vi "Scripting_RenameClassControlsOfClass.vi"(8 "error in (no error)":errorcluster, 10 "ClassControlName":string, 11 "LVClassLibrary in":refnum<vi>) -> (0 "error out":errorcluster)   [LabVIEW 2020, in "Scripting.lvclass"]
uses:
  <resource>/Framework/Providers/Open_GDS/ClassProviders/Common/ScriptingFunctions/Scripting.lvclass
  <vilib>/regexp/Match Regular Expression.xnode
panel:
  # "<ClassName> in/out\n<ClassName>\nobject in/out\nreference in/out"
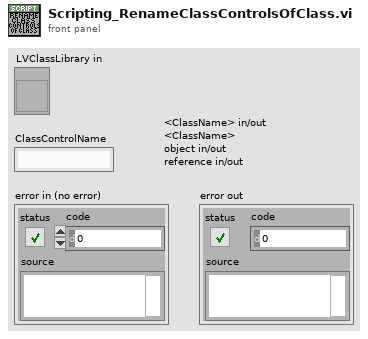
[diagram p1: front panel]
types:
  T1 = enum32{"invalid VI type", "Standard VI", "Control VI", "Global VI", "Polymorphic VI", "Configuration VI", "SubSystem", "Facade VI", "Method VI", "Statechart Diagram VI"}
  T2 = typedef "LVRectTypeDef.ctl" = cluster{"Left":i16, "Top":i16, "Right":i16, "Bottom":i16}
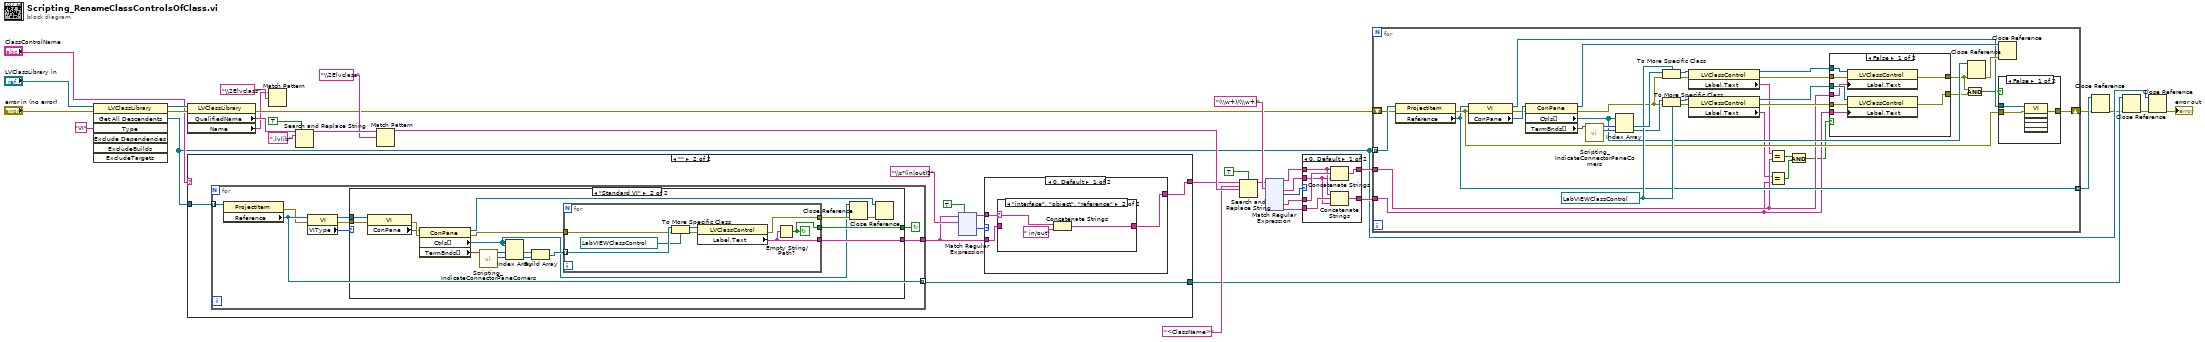
[diagram p0: block diagram]
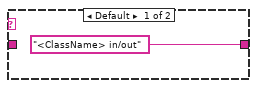
[diagram p3: hidden frame]
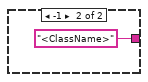
[diagram p4: hidden frame]
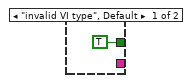
[diagram p5: hidden frame]
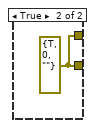
[diagram p7: hidden frame]
diagram:
  n1 = invoke class="LVClassLibrary" method="Get All Descendents"(reference="LVClassLibrary in", error in="error in (no error)", "Type"="VI") -> (reference out=w32:refnum<vi>, error out=w12:errorcluster, "All Descendents"=w8:refnum<vi>[])  [unwired: 4 in, 4 out]
  n2 = property class="LVClassLibrary"(reference=w32, error in=w12) -> (error out=w11:errorcluster, "QualifiedName"=w29:string, "Name"=w1:string)  [unwired: 1 out]
  n3 = case shown="\"\"" "ClassControlName" {
    selector: "ClassControlName" -> [w35 _]
    tunnel: [w35 w39] -> w9
    tunnel: w8 -> [_ w43]
    tunnel: [_ w42] -> w5
    frame Default {
    }
    frame "" {
      n4 = for {
        tunnel: w43 -> [w173] mode=indexing
        tunnel: [w172] -> w36
        tunnel: [w170] -> w42 mode=indexing
        stop <- w171 continue-if-true
        n5 = property class="ProjectItem"(reference=w173) -> (error out=w168:errorcluster, "Reference"=w170:refnum<vi>)  [unwired: 1 in, 1 out]
        n6 = property class="VI"(reference=w170, error in=w168) -> (reference out=w169:refnum<vi>, error out=w167:errorcluster, "VIType"=w166:T1)
        n7 = case shown="\"Standard VI\"" w166 {
          tunnel: [_ w182] -> w172
          tunnel: [TRUE w181] -> w171
          tunnel: w169 -> [_ w176]
          tunnel: w167 -> [_ w175]
          frame "invalid VI type", Default {
          }
          frame "Standard VI" {
            n8 = property class="VI"(reference=w176, error in=w175) -> (error out=w191:errorcluster, "ConPane"=w187:refnum<vi>)  [unwired: 1 out]
            n9 = property class="ConPane"(reference=w187, error in=w191) -> (reference out=w177:refnum<vi>, error out=w183:errorcluster, "Ctrls[]"=w179:refnum<vi>[], "TermBnds[]"=w188:T2[])
            n10 = call <resource>:"Scripting_IndicateConnectorPaneCorners.vi"("TermBnds[]"=w188) -> ("RightTop"=w190:i32, "LeftTop"=w189:i32)  [unwired: 7 in, 2 out]
            n11 = Index Array(array=w179, index #1=w189, index #2=w190) -> (element #1=w186:refnum<vi>, element #2=w185:refnum<vi>)
            n12 = Build Array(w186, w185) -> (w184:refnum<vi>[])
            n13 = for {
              tunnel: w184 -> [w199] mode=indexing
              tunnel: w183 -> [w196]
              tunnel: [w194] -> w182
              tunnel: [w193] -> w181
              tunnel: [w192] -> w180
              stop <- w193 continue-if-true
              n14 = To More Specific Class(target class=refnum<vi> refnum ("Other Refnum"), reference=w199, error in=w196) -> (specific class reference=w197:refnum<vi>, error out=w195:errorcluster)
              n15 = property class="LVClassControl"(reference=w197, error in=w195) -> (error out=w192:errorcluster, "Label.Text"=w194:string)  [unwired: 1 out]
              n16 = Empty String/Path?(string/path=w194) -> (empty?=w193:bool)
            }
            n17 = Close Reference(reference=w179, error in (no error)=w180) -> (error out=w178:errorcluster)
            n18 = Close Reference(reference=w177, error in (no error)=w178) -> ()  [unwired: 1 out]
          }
        }
      }
      n19 = xnode "Match Regular Expression"("input string"=w36, "regular expression"="\\s*(in|out)$", "ignore case? (F)"=TRUE) -> ("before match"=w38:string, "offset past match"=w40:i32)  [unwired: 3 in, 3 out]
      n20 = case shown="0, Default" w40 {
        tunnel: [w45 "<ClassName>" ("substring (\"\")")] -> w39
        tunnel: w38 -> [w46 _]
        tunnel: w36 -> [w44 _]
        frame 0, Default {
          n21 = case shown="\"interface\", \"object\", \"reference\"" w46 {
            selector: w46 -> [_ w48]
            tunnel: ["<ClassName> in/out" ("substring (\"\")") w50] -> w45
            tunnel: w44 -> [_ _]
            frame Default {
            }
            frame "interface", "object", "reference" {
              n22 = Concatenate Strings(w48, " in/out" ("string")) -> (w50:string)
            }
          }
        }
        frame -1 {
        }
      }
    }
  }
  n23 = Match Pattern(string=w1, regular expression="\\2Elvclass") -> ()  [unwired: 1 in, 4 out]
  n24 = Search and Replace String(replace all?=TRUE ("replace all? (F)"), input string=w29, search string=".lvlib" ("regular expression")) -> (result string=w33:string)  [unwired: 5 in, 3 out]
  n25 = Match Pattern(string=w33, regular expression="\\2Elvclass") -> (before substring=w34:string)  [unwired: 1 in, 3 out]
  n26 = Search and Replace String(case sensitive?=TRUE ("ignore case? (F)"), input string=w9, search string="<ClassName>" ("substring (\"\")"), replace string=w34) -> (result string=w18:string)  [unwired: 4 in, 3 out]
  n27 = xnode "Match Regular Expression"("input string"=w18, "regular expression"="(\\w+)/(\\w+)") -> ("before match"=w21:string, "after match"=w23:string, "offset past match"=w20:i32, "submatch 1"=w22:string, "submatch 2"=w24:string)  [unwired: 4 in, 2 out]
  n28 = case shown="0, Default" w20 {
    tunnel: w21 -> [w204 w206]
    tunnel: w22 -> [w205 _]
    tunnel: w23 -> [w202 _]
    tunnel: w24 -> [w203 _]
    tunnel: [w201 w206] -> w26
    tunnel: [w200 w206] -> w27
    frame 0, Default {
      n29 = Concatenate Strings(w204, w205, w202) -> (w201:string)
      n30 = Concatenate Strings(w204, w203, w202) -> (w200:string)
    }
    frame -1 {
    }
  }
  n31 = for {
    tunnel: w8 -> [w242] mode=indexing
    shift-right: [w221] -> w6
    shift-left: w11 -> [w241]
    tunnel: w26 -> [w212]
    tunnel: w27 -> [w210]
    tunnel: [w220] -> w7 mode=indexing
    w232 = refnum<vi> refnum ("Other Refnum")
    n32 = property class="ProjectItem"(reference=w242, error in=w241) -> (error out=w222:errorcluster, "Reference"=w220:refnum<vi>)  [unwired: 1 out]
    n33 = property class="VI"(reference=w220, error in=w222) -> (reference out=w224:refnum<vi>, error out=w227:errorcluster, "ConPane"=w239:refnum<vi>)
    n34 = property class="ConPane"(reference=w239, error in=w227) -> (reference out=w228:refnum<vi>, error out=w230:errorcluster, "Ctrls[]"=w229:refnum<vi>[], "TermBnds[]"=w238:T2[])
    n35 = call <resource>:"Scripting_IndicateConnectorPaneCorners.vi"("TermBnds[]"=w238) -> ("RightTop"=w236:i32, "LeftTop"=w237:i32)  [unwired: 7 in, 2 out]
    n36 = Index Array(array=w229, index #1=w237, index #2=w236) -> (element #1=w234:refnum<vi>, element #2=w231:refnum<vi>)
    n37 = To More Specific Class(target class=w232, reference=w234, error in=w230) -> (specific class reference=w218:refnum<vi>, error out=w235:errorcluster)
    n38 = To More Specific Class(target class=w232, reference=w231, error in=w230) -> (specific class reference=w215:refnum<vi>, error out=w233:errorcluster)
    n39 = property class="LVClassControl"(reference=w218, error in=w235) -> (reference out=w217:refnum<vi>, error out=w219:errorcluster, "Label.Text"=w213:string)
    n40 = property class="LVClassControl"(reference=w215, error in=w233) -> (reference out=w214:refnum<vi>, error out=w216:errorcluster, "Label.Text"=w211:string)
    n41 = Equal?(x=w213, y=w212) -> (x = y?=w209:bool)
    n42 = Equal?(x=w211, y=w210) -> (x = y?=w208:bool)
    n43 = And(x=w209, y=w208) -> (x .and. y?=w207:bool)
    n44 = case shown="False" w207 {
      tunnel: [w250 w251] -> w226
      tunnel: [w249 w251] -> w225
      tunnel: w219 -> [w248 _]
      tunnel: w217 -> [w247 _]
      tunnel: w216 -> [w246 _]
      tunnel: w214 -> [w245 _]
      tunnel: w212 -> [w244 _]
      tunnel: w210 -> [w243 _]
      frame False {
        n45 = property class="LVClassControl"(reference=w247, error in=w248, "Label.Text"=w244) -> (error out=w250:errorcluster)  [unwired: 1 out]
        n46 = property class="LVClassControl"(reference=w245, error in=w246, "Label.Text"=w243) -> (error out=w249:errorcluster)  [unwired: 1 out]
      }
      frame True {
        w251 = errorcluster {"status"=TRUE, "code"=0, "source"=""} ("error out")
      }
    }
    n47 = And(x=w226, y=w225) -> (x .and. y?=w223:bool)
    n48 = Close Reference(reference=w229, error in (no error)=w226) -> (error out=w240:errorcluster)
    n49 = Close Reference(reference=w228, error in (no error)=w240) -> ()  [unwired: 1 out]
    n50 = case shown="False" w223 {
      tunnel: w224 -> [w254 _]
      tunnel: w222 -> [w253 w255]
      tunnel: [w252 w255] -> w221
      frame False {
        n51 = invoke class="VI" method="Save.Instrument"(reference=w254, error in=w253) -> (error out=w252:errorcluster)  [unwired: 4 in, 5 out]
      }
      frame True {
      }
    }
  }
  n52 = Close Reference(reference=w7, error in (no error)=w6) -> (error out=w4:errorcluster)
  n53 = Close Reference(reference=w5, error in (no error)=w4) -> (error out=w3:errorcluster)
  n54 = Close Reference(reference=w8, error in (no error)=w3) -> (error out=→"error out":errorcluster)
